vi "Configure Calibration Alert Date.vi"(0 "VISA resource name":refnum<visa-resource-name>, 5 "Day (01)":i32=1 format="%02d", 7 "Month (01)":i32=1 format="%02d", 9 "Year (15)":i32=15 format="%02d", 11 "error IO":errorcluster) -> (4 "VISA resource Out":refnum<visa-resource-name>, 15 "error Out":errorcluster)   [LabVIEW 2020, in "eec EST 300.lvlib"]
doc: "Sets the Calibration Alert Date. The date is parsed out into 2 digit Day, 2 digit Month, 2 digit Year.\n\nThe Alert Date is like an alarm clock that will warn you in advance of the actual calibration due date. After a calibration is performed the Alert Date is automatically set 11 months after the calibration date."
uses:
  <instrlib>/eec EST 300/eec EST 300.lvlib
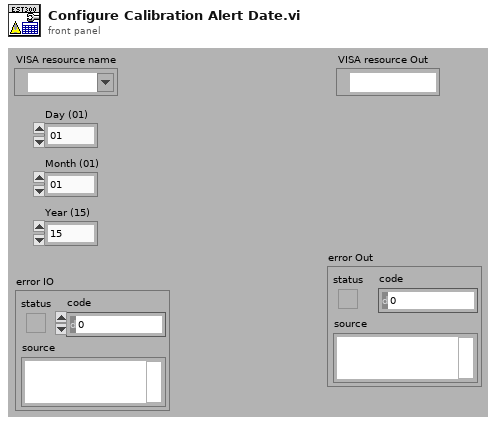
[diagram p1: front panel]
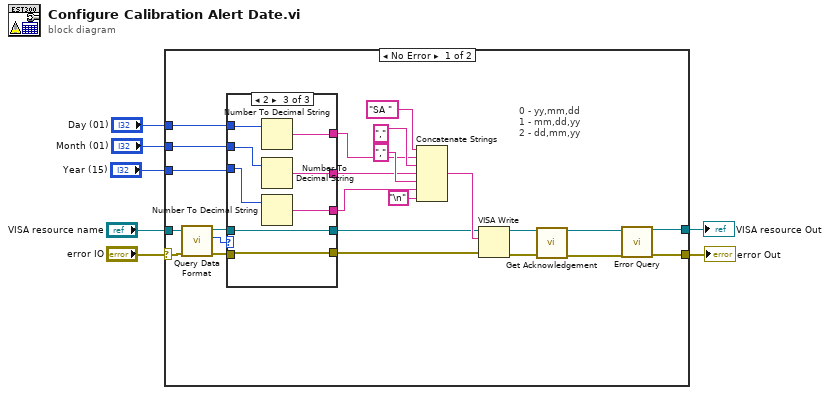
[diagram p0: block diagram]
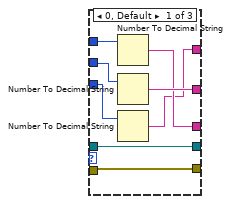
[diagram p2: hidden frame]
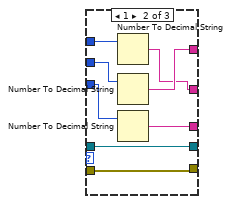
[diagram p3: hidden frame]
diagram:
  n1 = case shown="No Error" "error IO" {
    selector: "error IO" -> [w12 w57]
    tunnel: [w30 w57] -> w4
    tunnel: [w31 w56] -> w5
    tunnel: "VISA resource name" -> [w8 w56]
    tunnel: "Day (01)" -> [w16 _]
    tunnel: "Month (01)" -> [w15 _]
    tunnel: "Year (15)" -> [w14 _]
    frame No Error {
      # "0 - yy,mm,dd\n1 - mm,dd,yy\n2 - dd,mm,yy"
      n2 = call <instrlib>:"Query Data Format.vi"("error IO"=w12, "VISA resource name"=w8) -> ("error Out"=w11:errorcluster, "Date Format"=w9:u16, "VISA resource Out"=w10:refnum<visa-resource-name>)  [unwired: 7 in]
      n3 = case shown="2" w9 {
        tunnel: w16 -> [w39 w47 w55]
        tunnel: w15 -> [w38 w46 w54]
        tunnel: w14 -> [w37 w45 w53]
        tunnel: [w34 w43 w52] -> w21
        tunnel: [w36 w42 w51] -> w22
        tunnel: [w35 w44 w50] -> w23
        tunnel: [w33 w41 w49] -> w18
        tunnel: w10 -> [w33 w41 w49]
        tunnel: [w32 w40 w48] -> w17
        tunnel: w11 -> [w32 w40 w48]
        frame 0, Default {
          n4 = Number To Decimal String(number=w39) -> (decimal integer string=w35:string)  [unwired: 1 in]
          n5 = Number To Decimal String(number=w38) -> (decimal integer string=w36:string)  [unwired: 1 in]
          n6 = Number To Decimal String(number=w37) -> (decimal integer string=w34:string)  [unwired: 1 in]
        }
        frame 1 {
          n7 = Number To Decimal String(number=w47) -> (decimal integer string=w42:string)  [unwired: 1 in]
          n8 = Number To Decimal String(number=w46) -> (decimal integer string=w43:string)  [unwired: 1 in]
          n9 = Number To Decimal String(number=w45) -> (decimal integer string=w44:string)  [unwired: 1 in]
        }
        frame 2 {
          n10 = Number To Decimal String(number=w55) -> (decimal integer string=w52:string)  [unwired: 1 in]
          n11 = Number To Decimal String(number=w54) -> (decimal integer string=w51:string)  [unwired: 1 in]
          n12 = Number To Decimal String(number=w53) -> (decimal integer string=w50:string)  [unwired: 1 in]
        }
      }
      n13 = Concatenate Strings("SA " ("Command to Send (empty)"), w21, ",", w22, ",", w23, "\n") -> (w19:string)
      n14 = VISA Write(VISA resource name=w18, write buffer=w19, error in (no error)=w17) -> (VISA resource name out=w27:refnum<visa-resource-name>, error out=w26:errorcluster)  [unwired: 1 out]
      n15 = call <instrlib>:"Get Acknowledgement.vi"("VISA resource name"=w27, "error in (no error)"=w26) -> ("VISA resource name out"=w29:refnum<visa-resource-name>, "error out"=w28:errorcluster)  [unwired: 12 in]
      n16 = call <instrlib>:"Error Query.vi"("VISA resource name"=w29, "error in (no error)"=w28) -> ("VISA resource name out"=w31:refnum<visa-resource-name>, "error out"=w30:errorcluster)  [unwired: 10 in, 2 out]
    }
    frame Error {
    }
  }
  "VISA resource Out" <- w5
  "error Out" <- w4
